vi "运维调试_其他.vi"() -> ()   [LabVIEW 2016, in "其他.lvlib"]
uses:
  <vilib>/Utility/miscctls.llb/LVPointTypeDef.ctl
  <vilib>/ptbypt/NI_PtbyPt.lvlib
  <vilib>/Utility/config.llb/NI_LVConfig.lvlib
panel:
  out "最近一次启动时间":timestamp
  in  "跨度核查":bool
  in  "零点核查":bool
  in  "水样测试":bool
  in  "运行周期":T1={"运行模式"=enum."维护模式", "质控频次"=enum."关闭", "空白核查时间"=2, "跨度核查时间"=6, "多参数测试间隔"=4, "湿化学测试间隔"=4} {"多参数测试间隔" format="%.0f 分钟"; "湿化学测试间隔" format="%.0f 分钟"; "跨度核查时间" items=["00H", "01H", "02H", "03H", "04H", "05H", "06H", "07H", "08H", "09H", "10H", "11H", "12H", "13H", "14H", "15H", "16H", "17H", "18H", "19H", "20H", "21H", "22H", "23H", "关闭"]; "空白核查时间" items=["00H", "01H", "02H", "03H", "04H", "05H", "06H", "07H", "08H", "09H", "10H", "11H", "12H", "13H", "14H", "15H", "16H", "17H", "18H", "19H", "20H", "21H", "22H", "23H", "关闭"]}
  in  "模块启用设置":bool
  in  "站点信息设置":bool
  in  "定时重启":bool
  in  "首页设置":bool
  in  "短信报警设置":bool
  in  "布尔":bool
  # "多参数测试间隔："
  # "湿化学测试间隔："
  # "质控频次："
  # "运行模式："
  # "跨度核查时间："
  # "零点核查时间："
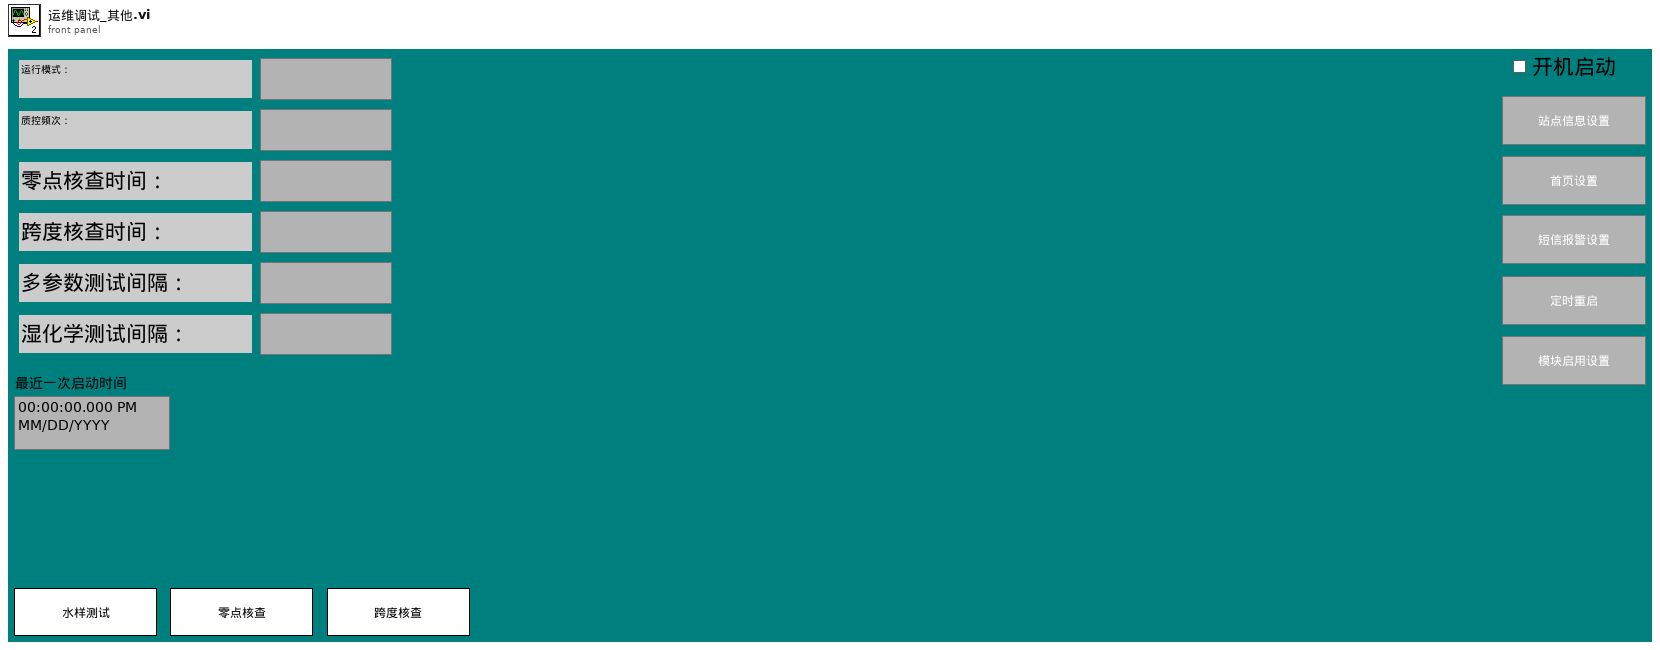
[diagram p1: front panel]
types:
  T1 = cluster{"运行模式":enum16{"维护模式", "常规模式", "应急模式", "质控模式"}, "质控频次":enum16{"关闭", "每天", "星期一", "星期二", "星期三", "星期四", "星期五", "星期六", "星期日"}, "空白核查时间":u16, "跨度核查时间":u16, "多参数测试间隔":u16, "湿化学测试间隔":u16}
  T2 = enum16{"启动测量", "标样核查", "零点核查", "跨度核查", "空白测试", "平行样测试", "加标回收", "空白校准", "标样校准", "初始化（清洗）", "停止测试", "仪器重启", "校时", "模式设置", "测量间隔设置"}
  T3 = cluster{"测试模式":enum16{"水样测试", "平行样测试", "集成干预测试", "加标回收"}, "参数启用":cluster{"多参数":bool, "湿化学":bool}}
  T4 = typedef "LVPointTypeDef.ctl" = cluster{"Horizontal":i16, "Vertical":i16}
  T5 = cluster{"频次":enum16{"关闭", "每天", "星期一", "星期二", "星期三", "星期四", "星期五", "星期六", "星期日"}, "时":u16, "分":u16}
  T6 = typedef "LVDateTimeRec.ctl" = cluster{"秒数的小数部分":dbl, "秒":i32, "分":i32, "时":i32, "日":i32, "月":i32, "年":i32, "天数（周）":i32, "天数（年）":i32, "DST":i32}
  T7 = enum16{"关闭", "每天", "星期一", "星期二", "星期三", "星期四", "星期五", "星期六", "星期日"}
  T8 = cluster{"运行模式":enum16{"维护模式", "常规模式", "应急模式", "质控模式"}, "质控频次":enum16{"关闭", "每天", "星期一", "星期二", "星期三", "星期四", "星期五", "星期六", "星期日"}, "空白核查时间":u16, "跨度核查时间":u16, "测量间隔":u16}
  T9 = enum32{"Bad", "Idle", "Run top level", "Running"}
  T10 = enum32{"Invalid", "Standard", "Closed", "Hidden", "Minimized", "Maximized"}
  T11 = typedef "NI_LVConfig.lvlib/Config Data RefNum.ctl" = refnum<k1>
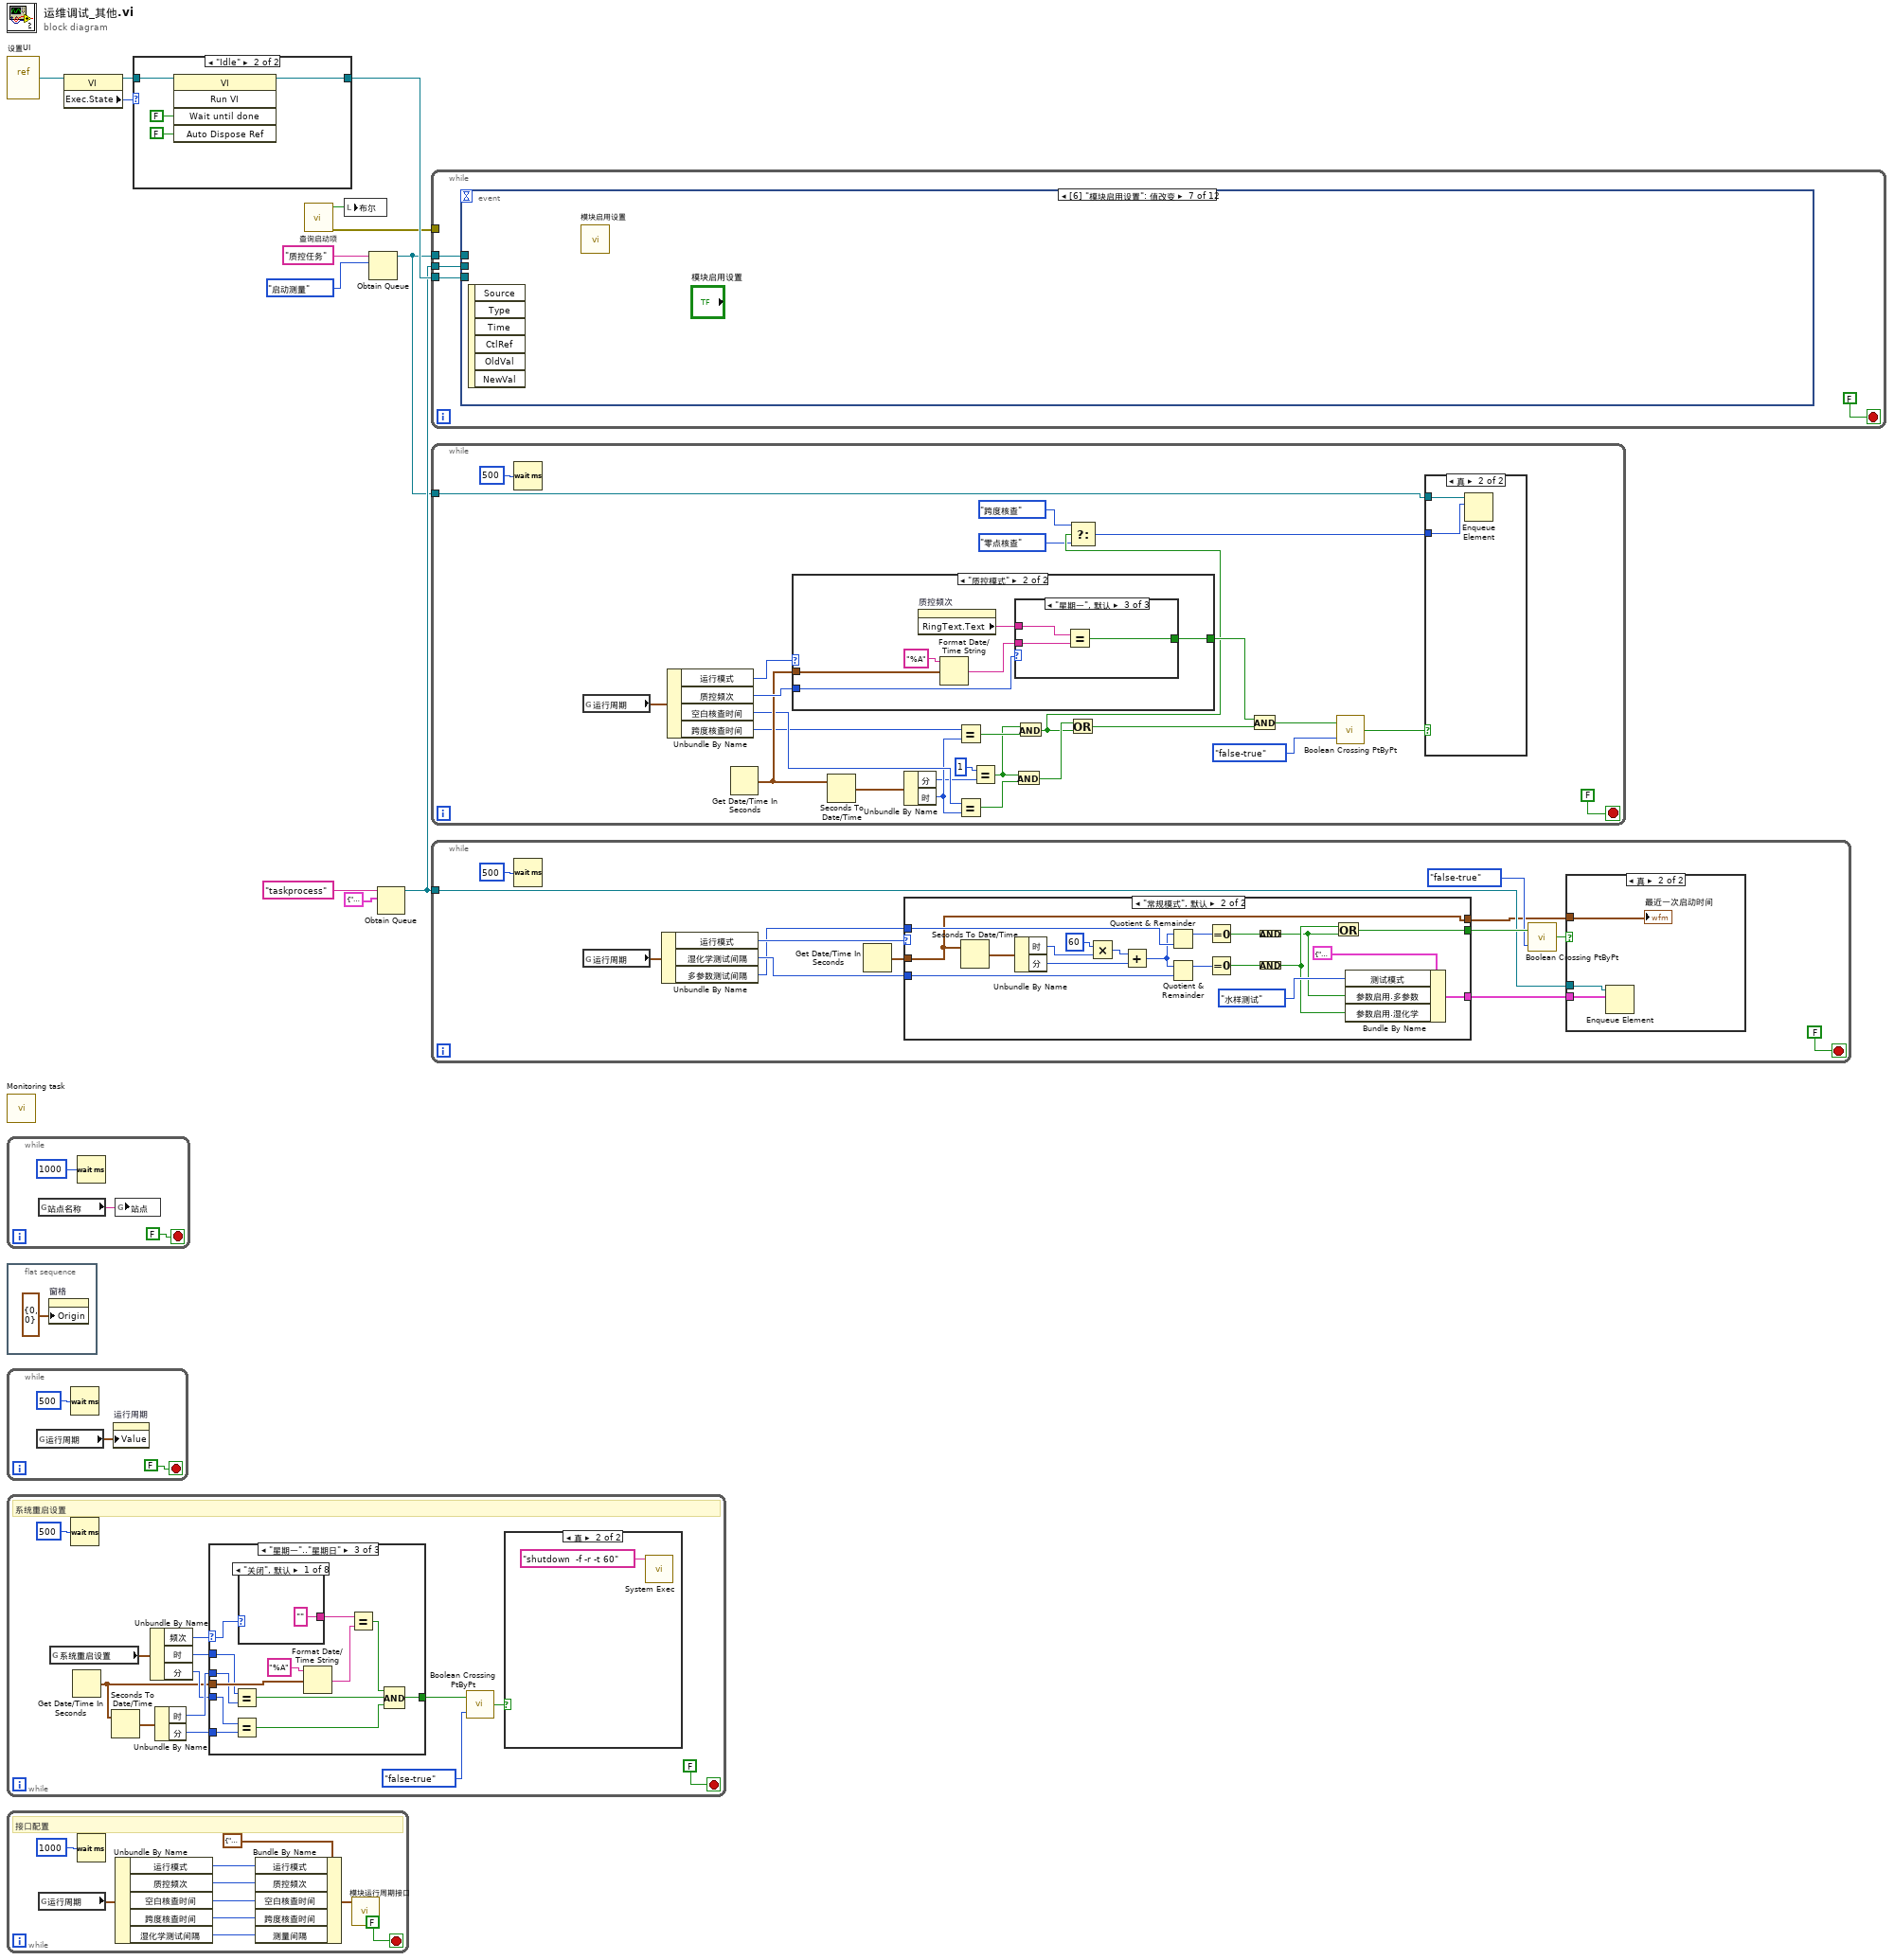
[diagram p0: block diagram]
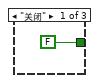
[diagram p4: hidden frame]
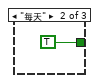
[diagram p5: hidden frame]
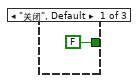
[diagram p9: hidden frame]
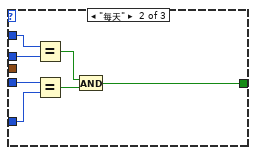
[diagram p10: hidden frame]
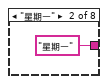
[diagram p11: hidden frame]
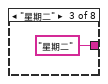
[diagram p12: hidden frame]
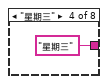
[diagram p13: hidden frame]
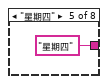
[diagram p14: hidden frame]
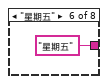
[diagram p15: hidden frame]
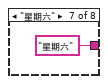
[diagram p16: hidden frame]
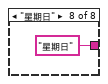
[diagram p17: hidden frame]
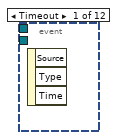
[diagram p19: hidden frame]
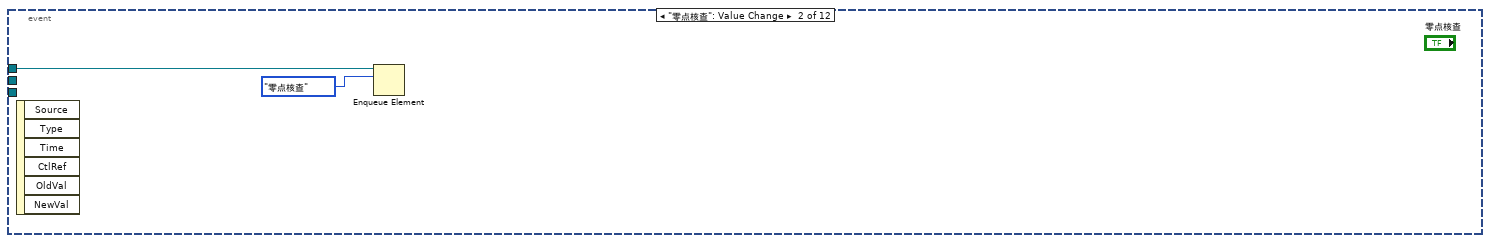
[diagram p20: hidden frame]
diagram:
  n1 = vi-ref "设置UI.vi"() -> (w10:refnum<vi>)
  n2 = call "Monitoring task.vi"() -> ()  [unwired: 12 in]
  n3 = while {
    stop <- FALSE stop-if-true
    n4 = global read "系统设置全局变量.vi" "站点名称"() -> (w13:string)
    n5 = Wait (ms)(milliseconds to wait=u32 1000 ("等待时间（毫秒）")) -> ()  [unwired: 1 out]
    n6 = global write "短信服务全局变量.vi" "站点"(w13) -> ()
  }
  n7 = flat-sequence {
    frame #0 {
      n8 = property on="窗格" class="Pane"("Origin"=T4 {"Horizontal"=0, "Vertical"=0} ("原点")) -> ()  [unwired: 2 in, 2 out]
    }
  }
  n9 = while {
    stop <- FALSE stop-if-true
    n10 = global read "系统设置全局变量.vi" "运行周期"() -> (w17:T1)
    n11 = Wait (ms)(milliseconds to wait=u32 500 ("等待时间（毫秒）")) -> ()  [unwired: 1 out]
    n12 = property on="运行周期" class="Clust (严格)"("Value"=w17) -> ()  [unwired: 2 in, 2 out]
  }
  n13 = while {
    stop <- FALSE stop-if-true
    # "系统重启设置"
    n14 = global read "系统设置全局变量.vi" "系统重启设置"() -> (w32:T5)
    n15 = Wait (ms)(milliseconds to wait=u32 500 ("等待时间（毫秒）")) -> ()  [unwired: 1 out]
    n16 = Get Date/Time In Seconds() -> (seconds since 1Jan1904=w23:timestamp)
    n17 = Seconds To Date/Time(time stamp (now)=w23) -> (date time rec=w30:T6)  [unwired: 1 in]
    n18 = Unbundle By Name(w32) -> ("频次"=w31:T7, "时"=w27:u16, "分"=w26:u16)
    n19 = Unbundle By Name(w30) -> ("时"=w29:i32, "分"=w28:i32)
    n20 = case shown="\"星期一\"..\"星期日\"" w31 {
      selector: w31 -> [_ _ w52]
      tunnel: [FALSE w35 w42] -> w22
      tunnel: w29 -> [_ w41 w46]
      tunnel: w28 -> [_ w38 w44]
      tunnel: w27 -> [_ w40 w47]
      tunnel: w26 -> [_ w39 w45]
      tunnel: w23 -> [_ _ w53]
      frame "关闭", Default {
      }
      frame "每天" {
        n21 = Equal?(x=w40, y=w41) -> (x = y?=w36:bool)
        n22 = Equal?(x=w39, y=w38) -> (x = y?=w37:bool)
        n23 = And(x=w36, y=w37) -> (x .and. y?=w35:bool)
      }
      frame "星期一".."星期日" {
        n24 = Equal?(x=w47, y=w46) -> (x = y?=w48:bool)
        n25 = Equal?(x=w45, y=w44) -> (x = y?=w49:bool)
        n26 = case shown="\"关闭\", 默认" w52 {
          tunnel: ["" ("时间格式字符串(%c)") "星期一" ("时间格式字符串(%c)") "星期二" ("时间格式字符串(%c)") "星期三" ("时间格式字符串(%c)") "星期四" ("时间格式字符串(%c)") "星期五" ("时间格式字符串(%c)") "星期六" ("时间格式字符串(%c)") "星期日" ("时间格式字符串(%c)")] -> w50
          frame "关闭", Default {
          }
          frame "星期一" {
          }
          frame "星期二" {
          }
          frame "星期三" {
          }
          frame "星期四" {
          }
          frame "星期五" {
          }
          frame "星期六" {
          }
          frame "星期日" {
          }
        }
        n27 = Format Date/Time String(time format string (%c)="%A" ("时间格式字符串(%c)"), seconds (now)=w53) -> (date/time string=w51:string)  [unwired: 1 in]
        n28 = Equal?(x=w50, y=w51) -> (x = y?=w43:bool)
        n29 = Compound Arithmetic op=AND ("复合运算")(w43, w48, w49) -> (w42:bool)
      }
    }
    n30 = call <vilib>:"Boolean Crossing PtByPt.vi"("direction"=enum16{"either", "false-true", "true-false"}."false-true", "input"=w22) -> ("crossing"=w20:bool)  [unwired: 1 in]
    n31 = case shown="真" w20 {
      frame False {
      }
      frame True {
        n32 = call <vilib>:"System Exec.vi"("command line"="shutdown  -f -r -t 60") -> ()  [unwired: 7 in, 4 out]
      }
    }
  }
  n33 = while {
    stop <- FALSE stop-if-true
    # "接口配置"
    n34 = global read "系统设置全局变量.vi" "运行周期"() -> (w68:T1)
    n35 = Wait (ms)(milliseconds to wait=u32 1000 ("等待时间（毫秒）")) -> ()  [unwired: 1 out]
    n36 = Unbundle By Name(w68) -> ("运行模式"=w67:enum16{"维护模式", "常规模式", "应急模式", "质控模式"}, "质控频次"=w66:T7, "空白核查时间"=w65:u16, "跨度核查时间"=w64:u16, "湿化学测试间隔"=w63:u16)
    n37 = Bundle By Name(cluster=T8 {"运行模式"=enum."维护模式", "质控频次"=enum."关闭", "空白核查时间"=2, "跨度核查时间"=6, "测量间隔"=240} ("运行周期"), "运行模式"=w67, "质控频次"=w66, "空白核查时间"=w65, "跨度核查时间"=w64, "测量间隔"=w63) -> (w69:T8)
    n38 = call "模块运行周期接口.vi"("运行周期"=w69) -> ()  [unwired: 11 in]
  }
  n39 = property class="VI"(reference=w10) -> (reference out=w11:refnum<vi>, "Exec.State"=w12:T9)  [unwired: 1 in, 1 out]
  n40 = case shown="\"Idle\"" w12 {
    tunnel: w11 -> [w73 w75]
    tunnel: [w73 w74] -> w9
    frame "Bad", Default {
    }
    frame "Idle" {
      n41 = invoke class="VI" method="Run VI"(reference=w75, "Wait until done"=FALSE ("结束前等待"), "Auto Dispose Ref"=FALSE ("自动销毁引用")) -> (reference out=w74:refnum<vi>)  [unwired: 2 in, 4 out]
    }
  }
  n42 = call "查询启动项.vi"() -> ("error out"=w7:errorcluster, "包含启动项"=w8:bool)  [unwired: 10 in]
  n43 = local write "布尔"(w8) -> ()
  n44 = Obtain Queue(name (unnamed)="质控任务" ("名称（未命名）"), element data type=T2."启动测量" ("控制命令")) -> (queue out=w1:refnum<queue>)  [unwired: 3 in, 2 out]
  n45 = Obtain Queue(name (unnamed)="taskprocess" ("名称（未命名）"), element data type=T3 {"测试模式"=enum."水样测试", "参数启用"={"多参数"=FALSE, "湿化学"=FALSE}} ("参数")) -> (queue out=w5:refnum<queue>)  [unwired: 3 in, 2 out]
  n46 = while {
    tunnel: w9 -> [w80]
    tunnel: w7 -> [_]
    tunnel: w5 -> [w79]
    tunnel: w1 -> [w78]
    stop <- FALSE stop-if-true
    n47 = event shown="[6] \"模块启用设置\": 值改变" {
      selector: _ -> [_ _ _ _ _ _ _ _ _ _ _ _]
      dyn-events: _ -> [_ _ _ _ _ _ _ _ _ _ _ _]
      timeout: _ -> [_ _ _ _ _ _ _ _ _ _ _ _]
      tunnel: w80 -> [_ _ _ _ _ _ _ _ _ w110 _ _]
      tunnel: w79 -> [_ _ _ _ w94 _ _ _ _ _ _ _]
      tunnel: w78 -> [_ w83 w85 _ _ _ _ _ _ _ _ _]
      event Timeout {
        n48 = event-data() -> ()  [unwired: 1 in, 3 out]
      }
      event "零点核查": Value Change {
        n49 = event-data() -> ()  [unwired: 1 in, 6 out]
        n50 = Enqueue Element(queue=w83, element=T2."零点核查" ("元素")) -> ()  [unwired: 2 in, 3 out]
      }
      event "跨度核查": Value Change {
        n51 = event-data() -> ()  [unwired: 1 in, 6 out]
        n52 = Enqueue Element(queue=w85, element=T2."跨度核查" ("元素")) -> ()  [unwired: 2 in, 3 out]
      }
      event "运行周期.多参数测试间隔", "运行周期.湿化学测试间隔": Mouse Down {
        n53 = event-data() -> ("CtlRef"=w89:refnum<vi>)  [unwired: 1 in]
        n54 = property class="DigNum (严格)"(reference=w89) -> (reference out=w87:refnum<vi>, "Value"=w88:u16)  [unwired: 1 in, 1 out]
        n55 = call "数字键盘.vi"("OldNumber"=w88) -> ("NewNumber"=w86:dbl)
        n56 = property class="DigNum (严格)"(reference=w87, "Val(Sgnl)"=w86) -> ()  [unwired: 1 in, 2 out]
      }
      event "水样测试": Value Change {
        w90 = TRUE ("参数启用.氨氮")
        n57 = event-data() -> ()  [unwired: 1 in, 6 out]
        n58 = Bundle By Name(cluster=T3 {"测试模式"=enum."水样测试", "参数启用"={"多参数"=FALSE, "湿化学"=FALSE}} ("参数"), "测试模式"=enum16{"水样测试", "平行样测试", "集成干预测试", "加标回收"}."水样测试", "参数启用.多参数"=w90, "参数启用.湿化学"=w90) -> (w91:T3)
        n59 = Enqueue Element(queue=w94, element=w91) -> ()  [unwired: 2 in, 3 out]
      }
      event "运行周期": Value Change {
        n60 = event-data() -> ()  [unwired: 1 in, 6 out]
        n61 = flat-sequence {
          frame #0 {
            n62 = global write "系统设置全局变量.vi" "运行周期"("运行周期") -> ()
          }
          frame #1 {
            n63 = call <vilib>:"Application Directory.vi"() -> ("Application Directory"=w109:path)
            n64 = Build Path(base path=w109, name or relative path="data\\sys.ini" ("名称或相对路径")) -> (appended path=w107:path)
            n65 = call <vilib>:"Open Config Data.vi"("configuration file path"=w107) -> ("error out"=w103:errorcluster, "refnum"=w106:T11)  [unwired: 8 in, 1 out]
            n66 = vi-ref "系统设置全局变量.vi"() -> (w105:refnum<vi>)
            n67 = call <userlib>:"Write Panel to INI__ogtk.vi"("error in (no error)"=w103, "VI ref"=w105, "refnum"=w106) -> ("error out"=w102:errorcluster, "refnum out"=w104:T11)  [unwired: 7 in]
            n68 = call <vilib>:"Close Config Data.vi"("error in (no error)"=w102, "refnum"=w104) -> ("error out"=w97:errorcluster, "file path"=w96:path)  [unwired: 8 in]
            n69 = Open/Create/Replace File(file path (use dialog)=w96, error in=w97) -> (refnum out=w100:refnum<file>, error out=w101:errorcluster)  [unwired: 4 in, 1 out]
            n70 = Flush File(refnum=w100, error in=w101) -> (refnum out=w99:refnum<file>, error out=w98:errorcluster)
            n71 = Close File(refnum=w99, error in=w98) -> ()  [unwired: 2 out]
          }
        }
      }
      event "模块启用设置": Value Change {
        n72 = event-data() -> ()  [unwired: 1 in, 6 out]
        n73 = call "模块启用设置.vi"() -> ()  [unwired: 12 in]
      }
      event "首页设置": Value Change {
        n74 = event-data() -> ()  [unwired: 1 in, 6 out]
        n75 = call "首页显示设置.vi"() -> ()  [unwired: 12 in]
      }
      event "定时重启": Value Change {
        n76 = event-data() -> ()  [unwired: 1 in, 6 out]
        n77 = call "重启设置.vi"() -> ()  [unwired: 12 in]
      }
      event "短信报警设置": Value Change {
        n78 = event-data() -> ()  [unwired: 1 in, 6 out]
        n79 = invoke class="VI" method="FP.Open"(reference=w110, "Activate"=TRUE ("激活？"), "State"=T10."Standard" ("状态")) -> ()  [unwired: 2 in, 5 out]
      }
      event "布尔": Value Change {
        n80 = event-data() -> ("NewVal"=w113:bool)  [unwired: 1 in, 5 out]
        n81 = case shown="真" w113 {
          tunnel: [w118 w123] -> _
          frame False {
            n82 = call "删除启动项.vi"() -> ("error out"=w118:errorcluster, "删除标记"=w117:bool)  [unwired: 10 in]
            n83 = Select(t="删除成功" ("消息"), s=w117, f="删除失败" ("消息")) -> (s? t:f=w116:string)
            n84 = One Button Dialog(message=w116) -> ()  [unwired: 1 in, 1 out]
          }
          frame True {
            n85 = call "添加启动项.vi"() -> ("error out"=w123:errorcluster, "添加成功标记"=w119:bool)  [unwired: 10 in]
            n86 = local write "布尔"(w119) -> ()
            n87 = Select(t="添加成功" ("消息"), s=w119, f="添加失败" ("消息")) -> (s? t:f=w120:string)
            n88 = One Button Dialog(message=w120) -> ()  [unwired: 1 in, 1 out]
          }
        }
      }
      event "站点信息设置": Value Change {
        n89 = event-data() -> ()  [unwired: 1 in, 6 out]
        n90 = call "站点信息设置.vi"() -> ()  [unwired: 12 in]
      }
    }
  }
  n91 = while {
    tunnel: w1 -> [w128]
    stop <- FALSE stop-if-true
    n92 = Wait (ms)(milliseconds to wait=u32 500 ("等待时间（毫秒）")) -> ()  [unwired: 1 out]
    n93 = global read "系统设置全局变量.vi" "运行周期"() -> (w147:T1)
    n94 = Unbundle By Name(w147) -> ("运行模式"=w145:enum16{"维护模式", "常规模式", "应急模式", "质控模式"}, "质控频次"=w146:T7, "空白核查时间"=w142:u16, "跨度核查时间"=w140:u16)
    n95 = Get Date/Time In Seconds() -> (seconds since 1Jan1904=w144:timestamp)
    n96 = case shown="\"质控模式\"" w145 {
      tunnel: w146 -> [_ w154]
      tunnel: w144 -> [_ w153]
      tunnel: [_ w152] -> w134
      frame "维护模式", Default {
      }
      frame "质控模式" {
        n97 = property on="质控频次" class="Enum (严格)"() -> ("RingText.Text"=w157:string)  [unwired: 2 in, 2 out]
        n98 = Format Date/Time String(time format string (%c)="%A" ("时间格式字符串(%c)"), seconds (now)=w153) -> (date/time string=w156:string)  [unwired: 1 in]
        n99 = case shown="\"星期一\", 默认" w154 {
          tunnel: w156 -> [_ _ w162]
          tunnel: [FALSE TRUE w161] -> w152
          tunnel: w157 -> [_ _ w160]
          frame "关闭" {
          }
          frame "每天" {
          }
          frame "星期一", Default {
            n100 = Equal?(x=w160, y=w162) -> (x = y?=w161:bool)
          }
        }
      }
    }
    n101 = Seconds To Date/Time(time stamp (now)=w144) -> (date time rec=w143:T6)  [unwired: 1 in]
    n102 = Unbundle By Name(w143) -> ("分"=w139:i32, "时"=w141:i32)
    n103 = Equal?(x=w140, y=w141) -> (x = y?=w137:bool)
    n104 = Equal?(x=w142, y=w141) -> (x = y?=w138:bool)
    n105 = Equal?(x=1, y=w139) -> (x = y?=w124:bool)
    n106 = And(x=w124, y=w138) -> (x .and. y?=w136:bool)
    n107 = And(x=w124, y=w137) -> (x .and. y?=w133:bool)
    n108 = Select(t=T2."跨度核查" ("控制命令"), s=w133, f=T2."零点核查" ("控制命令")) -> (s? t:f=w129:T2)
    n109 = Or(x=w136, y=w133) -> (x .or. y?=w135:bool)
    n110 = And(x=w134, y=w135) -> (x .and. y?=w130:bool)
    n111 = call <vilib>:"Boolean Crossing PtByPt.vi"("direction"=enum16{"either", "false-true", "true-false"}."false-true", "input"=w130) -> ("crossing"=w127:bool)  [unwired: 1 in]
    n112 = case shown="真" w127 {
      tunnel: w129 -> [_ w150]
      tunnel: w128 -> [_ w151]
      frame False {
      }
      frame True {
        n113 = Enqueue Element(queue=w151, element=w150) -> ()  [unwired: 2 in, 3 out]
      }
    }
  }
  n114 = while {
    tunnel: w5 -> [w168]
    stop <- FALSE stop-if-true
    n115 = Wait (ms)(milliseconds to wait=u32 500 ("等待时间（毫秒）")) -> ()  [unwired: 1 out]
    n116 = global read "系统设置全局变量.vi" "运行周期"() -> (w167:T1)
    n117 = Unbundle By Name(w167) -> ("运行模式"=w172:enum16{"维护模式", "常规模式", "应急模式", "质控模式"}, "湿化学测试间隔"=w173:u16, "多参数测试间隔"=w166:u16)
    n118 = Get Date/Time In Seconds() -> (seconds since 1Jan1904=w163:timestamp)
    n119 = case shown="\"常规模式\", 默认" w172 {
      tunnel: w163 -> [_ w180]
      tunnel: w173 -> [_ w183]
      tunnel: [_ w193] -> w171
      tunnel: w166 -> [_ w196]
      tunnel: [_ w194] -> w165
      tunnel: [_ w180] -> w164
      frame "维护模式" {
      }
      frame "常规模式", Default {
        n120 = Seconds To Date/Time(time stamp (now)=w180) -> (date time rec=w188:T6)  [unwired: 1 in]
        n121 = Unbundle By Name(w188) -> ("时"=w187:i32, "分"=w184:i32)
        n122 = Multiply(x=60, y=w187) -> (x*y=w185:i32)
        n123 = Add(x=w185, y=w184) -> (x+y=w181:i32)
        n124 = Quotient & Remainder(x=w181, y=w196) -> (x-y*floor(x/y)=w192:i32)  [unwired: 1 out]
        n125 = Quotient & Remainder(x=w181, y=w183) -> (x-y*floor(x/y)=w182:i32)  [unwired: 1 out]
        n126 = Equal To 0?(x=w192) -> (x = 0?=w195:bool)
        n127 = Equal To 0?(x=w182) -> (x = 0?=w197:bool)
        n128 = Compound Arithmetic op=AND ("复合运算")(w195) -> (w179:bool)
        n129 = Compound Arithmetic op=AND ("复合运算")(w197) -> (w189:bool)
        n130 = Or(x=w189, y=w179) -> (x .or. y?=w193:bool)
        n131 = Bundle By Name(cluster=T3 {"测试模式"=enum."水样测试", "参数启用"={"多参数"=FALSE, "湿化学"=FALSE}} ("参数"), "测试模式"=enum16{"水样测试", "平行样测试", "集成干预测试", "加标回收"}."水样测试", "参数启用.多参数"=w179, "参数启用.湿化学"=w189) -> (w194:T3)
      }
    }
    n132 = call <vilib>:"Boolean Crossing PtByPt.vi"("direction"=enum16{"either", "false-true", "true-false"}."false-true", "input"=w171) -> ("crossing"=w170:bool)  [unwired: 1 in]
    n133 = case shown="真" w170 {
      tunnel: w168 -> [_ w178]
      tunnel: w165 -> [_ w177]
      tunnel: w164 -> [_ w176]
      frame False {
      }
      frame True {
        n134 = Enqueue Element(queue=w178, element=w177) -> ()  [unwired: 2 in, 3 out]
        "最近一次启动时间" <- w176
      }
    }
  }
